vi "Generic_Control_Window.vi"() -> ()   [LabVIEW 2018]
uses:
  <vilib>/Utility/miscctls.llb/LVPointTypeDef.ctl
panel:
  out "String":string="DER0"
  in  "Close":bool
  in  "Set Control Mode":bool
  in  "Set Variable 2":bool
  in  "Variable 2 Setpoint":sgl
  in  "Set Variable 1":bool
  in  "Variable 1 Setpoint":sgl
  in  "Cotrol Mode":enum16{"Master", "Slave"}(ring)
  in  "DER Stop Button":bool
  in  "DER Start Button":bool
  out "DER":i32
  out "Commands Cluster":T1
  out "Event":refnum<user-event>
  out "DER Names":string[](array[string])
  # "Control"
  # "Device:"
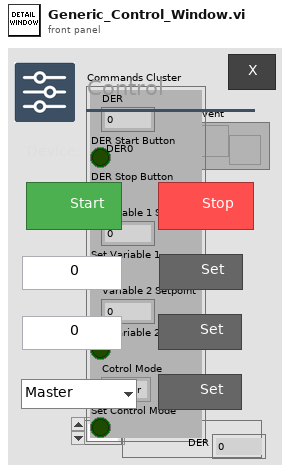
[diagram p1: front panel]
types:
  T1 = cluster{"DER":i32, "DER Start Button":bool, "DER Stop Button":bool, "Variable 1 Setpoint":dbl, "Set Variable 1":bool, "Variable 2 Setpoint":dbl, "Set Variable 2":bool, "Cotrol Mode":enum16{"Master", "Slave"}, "Set Control Mode":bool}
  T2 = typedef "LVPointTypeDef.ctl" = cluster{"Horizontal":i16, "Vertical":i16}
  T3 = enum32{"Invalid", "Default", "Floating", "Floating/Auto-Hide", "Modal"}
  T4 = cluster{"DER":i32, "DER Start Button":bool, "DER Stop Button":bool, "Variable 1 Setpoint":sgl, "Set Variable 1":bool, "Variable 2 Setpoint":sgl, "Set Variable 2":bool, "Cotrol Mode":enum16{"Master", "Slave"}, "Set Control Mode":bool}
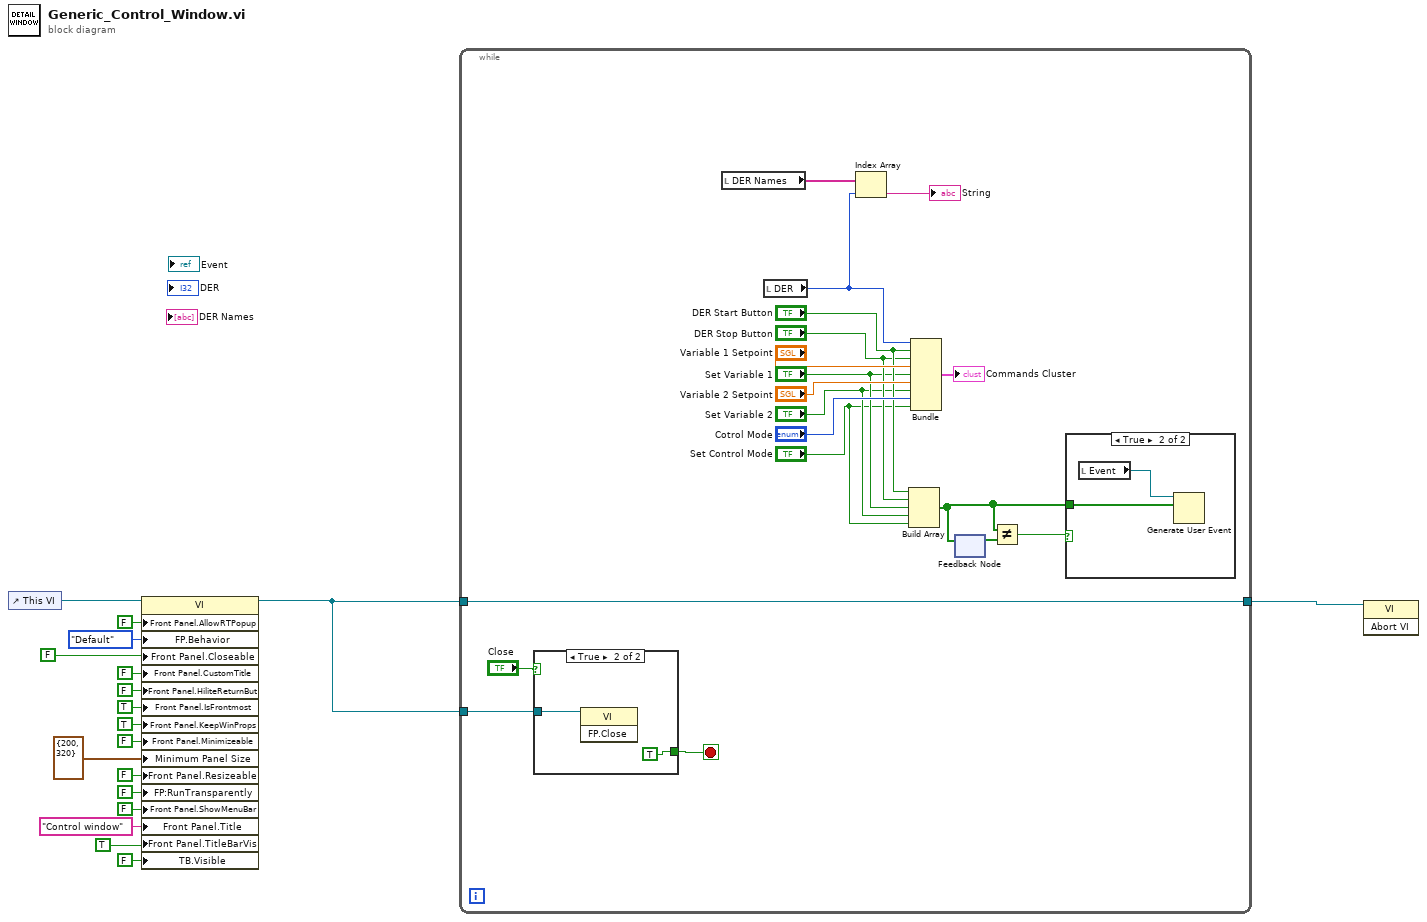
[diagram p0: block diagram]
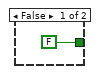
[diagram p3: hidden frame]
diagram:
  n1 = control-ref of="This VI"() -> (w18:refnum<vi>)
  n2 = property class="VI"(reference=w18, "Front Panel.AllowRTPopup"=FALSE ("Front Panel Window:Allow Runtime PopUp"), "FP.Behavior"=T3."Default" ("Front Panel Window:Behavior"), "Front Panel.Closeable"=FALSE ("Front Panel Window:Closeable"), "Front Panel.CustomTitle"=FALSE ("Front Panel Window:Custom Title"), "Front Panel.HiliteReturnBut"=FALSE ("Front Panel Window:Highlight Return Button"), "Front Panel.IsFrontmost"=TRUE ("Front Panel Window:Is Frontmost"), "Front Panel.KeepWinProps"=TRUE ("Front Panel Window:Keep Window Proportions"), "Front Panel.Minimizeable"=FALSE ("Front Panel Window:Minimizable"), "Minimum Panel Size"=T2 {"Horizontal"=200, "Vertical"=320} ("Front Panel Window:Minimum Size"), "Front Panel.Resizeable"=FALSE ("Front Panel Window:Resizable"), "FP:RunTransparently"=FALSE ("Front Panel Window:Run VI Transparently"), "Front Panel.ShowMenuBar"=FALSE ("Front Panel Window:Show Menu Bar"), "Front Panel.Title"="Control window" ("Front Panel Window:Title"), "Front Panel.TitleBarVis"=TRUE ("Front Panel Window:Title Bar Visible"), "TB.Visible"=FALSE ("Tool Bar:Visible")) -> (reference out=w2:refnum<vi>)  [unwired: 1 in, 1 out]
  n3 = while {
    tunnel: w2 -> [w36]
    tunnel: [w34] -> w1
    tunnel: w2 -> [w34]
    stop <- w35 stop-if-true
    n4 = case shown="True" "Close" {
      tunnel: w36 -> [_ w42]
      tunnel: [FALSE TRUE] -> w35
      frame False {
      }
      frame True {
        n5 = invoke class="VI" method="FP.Close"(reference=w42) -> ()  [unwired: 2 in, 3 out]
      }
    }
    n6 = local read "DER Names"() -> (w22:string[])
    n7 = local read "DER"() -> (w21:i32)
    n8 = Index Array(array=w22, index=w21) -> (element=→"String":string)
    n9 = Build Array("DER Start Button", "DER Stop Button", "Set Variable 1", "Set Variable 2", "Set Control Mode") -> (w26:bool[])
    n10 = Bundle("DER"=w21, "DER Start Button"="DER Start Button", "DER Stop Button"="DER Stop Button", "Variable 1 Setpoint"="Variable 1 Setpoint", "Set Variable 1"="Set Variable 1", "Variable 2 Setpoint"="Variable 2 Setpoint", "Set Variable 2"="Set Variable 2", "Cotrol Mode"="Cotrol Mode", "Set Control Mode"="Set Control Mode") -> (→"Commands Cluster":T4)  [unwired: 1 in]
    n11 = feedback-in #1(w26) -> ()
    n12 = feedback #1() -> (w27:bool[])  [unwired: 1 in]
    n13 = Not Equal?(x=w26, y=w27) -> (x != y?=w25:bool)
    n14 = case shown="True" w25 {
      tunnel: w26 -> [_ w38]
      frame False {
      }
      frame True {
        n15 = local read "Event"() -> (w39:refnum<user-event>)
        n16 = Generate User Event(user event=w39, event data cluster=w38) -> ()  [unwired: 2 in, 2 out]
      }
    }
  }
  n17 = invoke class="VI" method="Abort VI"(reference=w1) -> ()  [unwired: 2 in, 3 out]
